vi "WPI_CANTalonSRX_ConfigEnabledLimits.vi"(0 "CAN Talon SRX Ref":T1={"DeviceStatus"={"status"=FALSE, "code"=0, "source"=""}, "Type"=enum."PWM", "PWM"={"PWM Channel"=enum."PWM 1", "DeadBand"={"Name"="", "maxPositivePwm"=0, "minPositivePwm"=0, "centerPwm"=0, "maxNegativePwm"=0, "minNegativePwm"=0, "angularRange"=0}}, "CAN"={"Device Number"=0, "SetOutput VI Ref"=variant(enum8{"Percent VBus", "Current", "Speed", "Position", "Voltage"} enum."Percent VBus"), "GetOutput VI Ref"=variant(refnum<k1> refnum), "Enable VI Ref"=variant(dbl 12.0), "Disable VI Ref"=variant(enum8{"Percent VBus", "Speed", "Position", "Slave", "Unchanged / Invalid", "Voltage Compensation", "Current", "Motion Profile"} enum."Percent VBus"), "Data"=variant}, "Invert"=FALSE}, 5 "Override Limit Switches":bool, 7 "Forward Limit Switch Enable":bool=TRUE, 9 "Reverse Limit Switch Enable":bool=TRUE, 11 "error in (no error)":errorcluster, 12 "Forward Soft Limit Enable":bool, 13 "Reverse Soft Limit Enable":bool) -> (4 "CAN Talon SRX Ref":T1={"DeviceStatus"={"status"=FALSE, "code"=0, "source"=""}, "Type"=enum."PWM", "PWM"={"PWM Channel"=enum."PWM 1", "DeadBand"={"Name"="", "maxPositivePwm"=0, "minPositivePwm"=0, "centerPwm"=0, "maxNegativePwm"=0, "minNegativePwm"=0, "angularRange"=0}}, "CAN"={"Device Number"=0, "SetOutput VI Ref"=variant(enum8{"Percent VBus", "Current", "Speed", "Position", "Voltage"} enum."Percent VBus"), "GetOutput VI Ref"=variant(refnum<k1> refnum), "Enable VI Ref"=variant(dbl 12.0), "Disable VI Ref"=variant(enum8{"Percent VBus", "Speed", "Position", "Slave", "Unchanged / Invalid", "Voltage Compensation", "Current", "Motion Profile"} enum."Percent VBus"), "Data"=variant}, "Invert"=FALSE}, 15 "error out":errorcluster)   [LabVIEW 2016]
doc: "Configure the enable state of the hardware limit switches and the soft limits."
uses:
  <vilib>/Rock Robotics/WPI/MotorControl/WPI_MotorControlDeviceRef.ctl
  <vilib>/Rock Robotics/WPI/MotorControl/WPI_MotorControlType.ctl
  <vilib>/Rock Robotics/SystemInterfaces/DIO/FPGA_DIOPWMChannel.ctl
  <vilib>/Rock Robotics/WPI/PWM/WPI_PWMDeadband.ctl
  <vilib>/Rock Robotics/WPI/ThirdParty/CanMotor/TalonSRX/WPI_CANTalonSRX_GlobalOps.ctl
  <vilib>/Rock Robotics/WPI/ThirdParty/CanMotor/TalonSRX/WPI_CANTalonSRX_Params.ctl
  <vilib>/Rock Robotics/WPI/ThirdParty/CanMotor/TalonSRX/CTRE_CANTalonSRX_UsageTypes.ctl
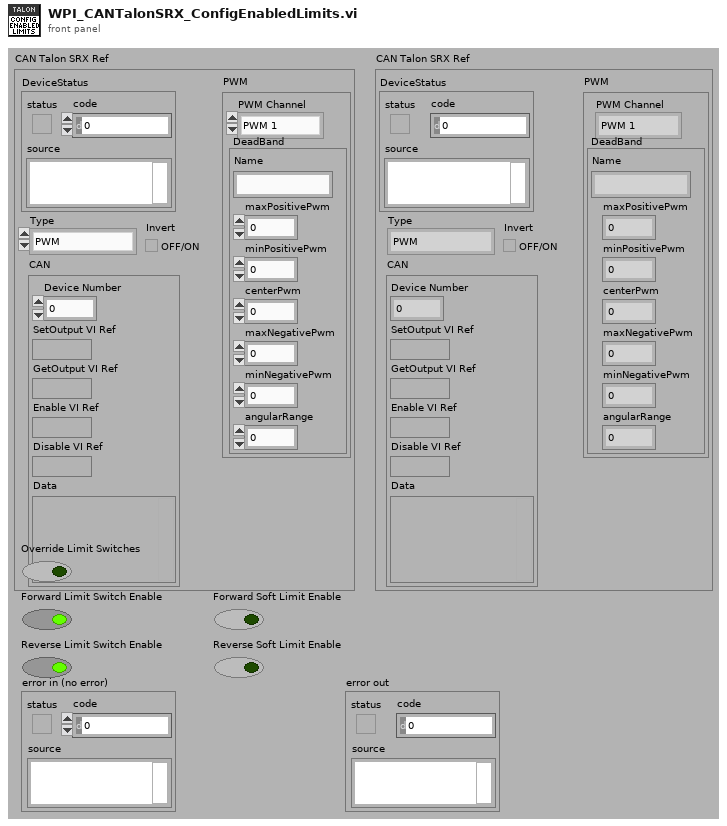
[diagram p1: front panel]
types:
  T1 = typedef "WPI_MotorControlDeviceRef.ctl" = cluster{"DeviceStatus":errorcluster, "Type":T2, "PWM":cluster{"PWM Channel":T3, "DeadBand":T4}, "CAN":cluster{"Device Number":u8, "SetOutput VI Ref":variant, "GetOutput VI Ref":variant, "Enable VI Ref":variant, "Disable VI Ref":variant, "Data":variant}, "Invert":bool}
  T2 = typedef "WPI_MotorControlType.ctl" = enum16{"PWM", "CAN"}
  T3 = typedef "FPGA_DIOPWMChannel.ctl" = enum8{"PWM 0", "PWM 1", "PWM 2", "PWM 3", "PWM 4", "PWM 5", "PWM 6", "PWM 7", "PWM 8", "PWM 9", "PWM MXP 0", "PWM MXP 1", "PWM MXP 2", "PWM MXP 3", "PWM MXP 4", "PWM MXP 5", "PWM MXP 6", "PWM MXP 7", "PWM MXP 8", "PWM MXP 9", "Invalid"}
  T4 = typedef "WPI_PWMDeadband.ctl" = cluster{"Name":string, "maxPositivePwm":i32, "minPositivePwm":i32, "centerPwm":i32, "maxNegativePwm":i32, "minNegativePwm":i32, "angularRange":u16}
  T5 = typedef "WPI_CANTalonSRX_GlobalOps.ctl" = enum16{"Read For Send", "Write After Receive General", "Write After Receive Feedback", "Write After Receive Encoder", "Write After Receive Ain", "Write Error", "Get All", "Set Output", "Set Mode", "Set Master ID", "Set Brake Mode", "Set Reverse Feedback Sensor", "Set Reverse Closed Loop Output", "Set Override Limits", "Set Forward Limit Enabled", "Set Reverse Limit Enabled", "Set Feedback Select", "Set Profile Select", "Set Throttle Ramp Rate", "Disable", "Set Enc Codes Per Rev", "Set Num Pot Turns", "Set Control Frame Rate", "Enable Legacy Control", "Write After Receive Pulse Width", "Set Enable Frame Rate", "Write After Receive Motion Profile", "Set Motion Profile Flow Control", "Set Motion Profile Control Frame Rate", "Set Current Limit Enable", "Set Usage Frame"}
  T6 = typedef "WPI_CANTalonSRX_Params.ctl" = u8
  T7 = typedef "CTRE_CANTalonSRX_UsageTypes.ctl" = u32
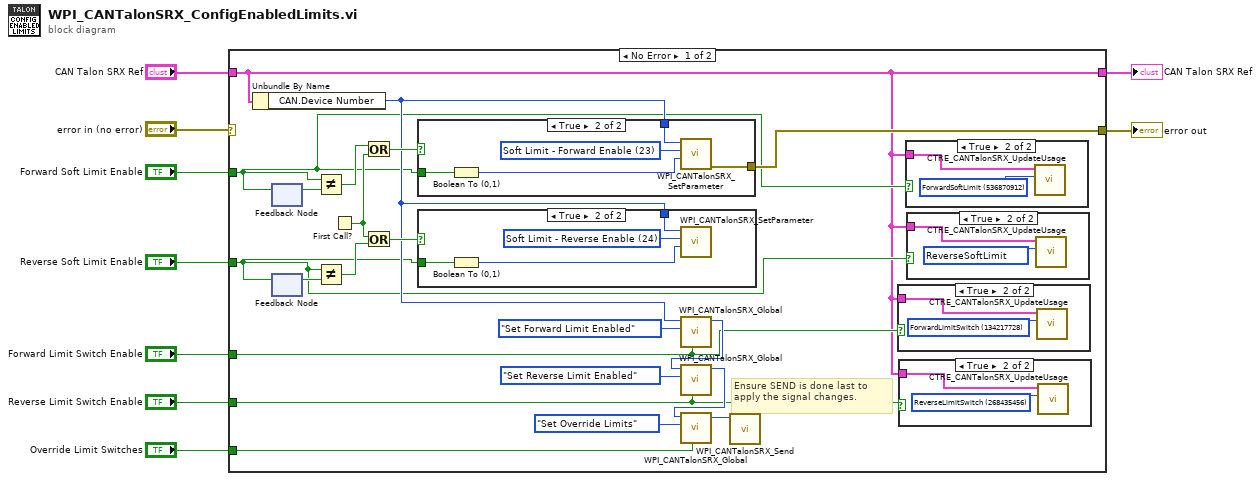
[diagram p0: block diagram]
diagram:
  n1 = case shown="No Error" "error in (no error)" {
    selector: "error in (no error)" -> [_ w49]
    tunnel: [w30 w49] -> w9
    tunnel: [w10 w48] -> w7
    tunnel: "CAN Talon SRX Ref" -> [w10 w48]
    tunnel: "Reverse Soft Limit Enable" -> [w13 _]
    tunnel: "Forward Soft Limit Enable" -> [w14 _]
    tunnel: "Reverse Limit Switch Enable" -> [w11 _]
    tunnel: "Forward Limit Switch Enable" -> [w12 _]
    tunnel: "Override Limit Switches" -> [w27 _]
    frame No Error {
      # "Ensure SEND is done last to apply the signal changes."
      n2 = Unbundle By Name(w10) -> ("CAN.Device Number"=w18:u8)
      n3 = feedback #1() -> (w21:bool)  [unwired: 1 in]
      n4 = feedback-in #1(w14) -> ()
      n5 = feedback-in #2(w13) -> ()
      n6 = feedback #2() -> (w25:bool)  [unwired: 1 in]
      n7 = Not Equal?(x=w14, y=w21) -> (x != y?=w22:bool)
      n8 = Not Equal?(x=w13, y=w25) -> (x != y?=w23:bool)
      n9 = First Call?() -> (First Call?: T/F=w20:bool)
      n10 = Or(x=w22, y=w20) -> (x .or. y?=w19:bool)
      n11 = Or(x=w20, y=w23) -> (x .or. y?=w24:bool)
      n12 = case shown="True" w19 {
        tunnel: w14 -> [_ w42]
        tunnel: [_ w40] -> w30
        tunnel: w18 -> [_ w39]
        frame False {
        }
        frame True {
          w43 = T6 23 items=["Slot 0 - P"=1, "Slot 0 - I"=2, "Slot 0 - D"=3, "Slot 0 - F"=4, "Slot 0 - I Zone"=5, "Slot 0 - Ramp Rate"=6, "Slot 1 - P"=11, "Slot 1 - I"=12, "Slot 1 - D"=13, "Slot 1 - F"=14, "Slot 1 - I Zone"=15, "Slot 1 - Ramp Rate"=16, "Soft Limit - Forward"=21, "Soft Limit - Reverse"=22, "Soft Limit - Forward Enable"=23, "Soft Limit - Reverse Enable"=24, "On Boot - Brake Mode"=31, "On Boot - Limit Normally Closed - Forward"=32, "On Boot - Limit Normally Closed - Reverse"=33, "On Boot - Limit Disabled - Forward"=34, "On Boot - Limit Disabled - Reverse"=35, "Fault - Over Temp"=41, "Fault - Under Voltage"=42, "Fault - Forward Limit"=43, "Fault - Reverse Limit"=44, "Fault - Hardware Failure"=45, "Fault - Forward Soft Limit"=46, "Fault - Reverse Soft Limit"=47, "Sticky Fault - Over Temp"=48, "Sticky Fault - Under Voltage"=49, "Sticky Fault - Forward Limit"=50, "Sticky Fault - Reverse Limit"=51, "Sticky Fault - Forward Soft Limit"=52, "Sticky Fault - Reverse Soft Limit"=53, "Applied Throttle"=61, "Closed-Loop Error"=62, "Select Feedback Device"=63, "Reverse Closed-Loop Output"=64, "Mode Select"=65, "Profile Slot Select"=66, "Ramp Throttle"=67, "Reverse Feedback Sensor"=68, "Limit Switch Enabled"=69, "Limit Switch Closed - Forward"=70, "Limit Switch Closed - Reverse"=71, "Sensor Position"=73, "Sensor Velocity"=74, "Current"=75, "Brake is Enabled"=76, "Encoder Position"=77, "Encoder Velocity"=78, "Encoder Index Rise Events"=79, "Encoder A Pin State"=80, "Encoder B Pin State"=81, "Encoder Index Pin State"=82, "Analog In with Overflow"=83, "Analog In Velocity"=84, "Temperature"=85, "Battery Voltage"=86, "Reset Count"=87, "Reset Flags"=88, "Firmware Version"=89, "Settings Changed"=90] ("Parameter")
          n13 = Boolean To (0,1)(Boolean=w42) -> (0, 1=w41:i16)
          n14 = call <vilib>:"WPI_CANTalonSRX_SetParameter.vi"("Value"=w41, "Parameter"=w43, "Device ID (0)"=w39) -> ("error out"=w40:errorcluster)  [unwired: 7 in, 1 out]
        }
      }
      n15 = case shown="True" w24 {
        tunnel: w13 -> [_ w46]
        tunnel: w18 -> [_ w44]
        frame False {
        }
        frame True {
          w47 = T6 24 items=["Slot 0 - P"=1, "Slot 0 - I"=2, "Slot 0 - D"=3, "Slot 0 - F"=4, "Slot 0 - I Zone"=5, "Slot 0 - Ramp Rate"=6, "Slot 1 - P"=11, "Slot 1 - I"=12, "Slot 1 - D"=13, "Slot 1 - F"=14, "Slot 1 - I Zone"=15, "Slot 1 - Ramp Rate"=16, "Soft Limit - Forward"=21, "Soft Limit - Reverse"=22, "Soft Limit - Forward Enable"=23, "Soft Limit - Reverse Enable"=24, "On Boot - Brake Mode"=31, "On Boot - Limit Normally Closed - Forward"=32, "On Boot - Limit Normally Closed - Reverse"=33, "On Boot - Limit Disabled - Forward"=34, "On Boot - Limit Disabled - Reverse"=35, "Fault - Over Temp"=41, "Fault - Under Voltage"=42, "Fault - Forward Limit"=43, "Fault - Reverse Limit"=44, "Fault - Hardware Failure"=45, "Fault - Forward Soft Limit"=46, "Fault - Reverse Soft Limit"=47, "Sticky Fault - Over Temp"=48, "Sticky Fault - Under Voltage"=49, "Sticky Fault - Forward Limit"=50, "Sticky Fault - Reverse Limit"=51, "Sticky Fault - Forward Soft Limit"=52, "Sticky Fault - Reverse Soft Limit"=53, "Applied Throttle"=61, "Closed-Loop Error"=62, "Select Feedback Device"=63, "Reverse Closed-Loop Output"=64, "Mode Select"=65, "Profile Slot Select"=66, "Ramp Throttle"=67, "Reverse Feedback Sensor"=68, "Limit Switch Enabled"=69, "Limit Switch Closed - Forward"=70, "Limit Switch Closed - Reverse"=71, "Sensor Position"=73, "Sensor Velocity"=74, "Current"=75, "Brake is Enabled"=76, "Encoder Position"=77, "Encoder Velocity"=78, "Encoder Index Rise Events"=79, "Encoder A Pin State"=80, "Encoder B Pin State"=81, "Encoder Index Pin State"=82, "Analog In with Overflow"=83, "Analog In Velocity"=84, "Temperature"=85, "Battery Voltage"=86, "Reset Count"=87, "Reset Flags"=88, "Firmware Version"=89, "Settings Changed"=90] ("Parameter")
          n16 = Boolean To (0,1)(Boolean=w46) -> (0, 1=w45:i16)
          n17 = call <vilib>:"WPI_CANTalonSRX_SetParameter.vi"("Value"=w45, "Parameter"=w47, "Device ID (0)"=w44) -> ()  [unwired: 7 in, 2 out]
        }
      }
      n18 = call <vilib>:"WPI_CANTalonSRX_Global.vi"("Set Boolean"=w12, "Operation"=WPI_CANTalonSRX_GlobalOps."Set Forward Limit Enabled", "Device ID (0)"=w18) -> ("Device ID Out"=w16:u8)  [unwired: 6 in, 2 out]
      n19 = call <vilib>:"WPI_CANTalonSRX_Global.vi"("Set Boolean"=w11, "Operation"=WPI_CANTalonSRX_GlobalOps."Set Reverse Limit Enabled", "Device ID (0)"=w16) -> ("Device ID Out"=w15:u8)  [unwired: 6 in, 2 out]
      n20 = call <vilib>:"WPI_CANTalonSRX_Global.vi"("Set Boolean"=w27, "Operation"=WPI_CANTalonSRX_GlobalOps."Set Override Limits", "Device ID (0)"=w15) -> ("Device ID Out"=w17:u8)  [unwired: 6 in, 2 out]
      n21 = call <vilib>:"WPI_CANTalonSRX_Send.vi"("Device ID (0)"=w17) -> ()  [unwired: 10 in, 1 out]
      n22 = case shown="True" w12 {
        tunnel: w10 -> [_ w34]
        frame False {
        }
        frame True {
          w33 = T7 134217728 items=["Default"=0, "PercentVbus"=1, "Position"=2, "Speed"=4, "Current"=8, "Voltage"=16, "Follower"=32, "MotionProfile"=64, "MotionMagic"=128, "VRampRate"=4194304, "CurrentLimit"=8388608, "ZeroSensorI"=16777216, "ZeroSensorF"=33554432, "ZeroSensorR"=67108864, "ForwardLimitSwitch"=134217728, "ReverseLimitSwitch"=268435456, "ForwardSoftLimit"=536870912, "ReverseSoftLimit"=1073741824, "MultiProfile"=2147483648] ("Usage")
          n23 = call <vilib>:"CTRE_CANTalonSRX_UpdateUsage.vi"("Usage"=w33, "CAN Talon SRX Ref"=w34) -> ()  [unwired: 10 in]
        }
      }
      n24 = case shown="True" w11 {
        tunnel: w10 -> [_ w32]
        frame False {
        }
        frame True {
          w31 = T7 268435456 items=["Default"=0, "PercentVbus"=1, "Position"=2, "Speed"=4, "Current"=8, "Voltage"=16, "Follower"=32, "MotionProfile"=64, "MotionMagic"=128, "VRampRate"=4194304, "CurrentLimit"=8388608, "ZeroSensorI"=16777216, "ZeroSensorF"=33554432, "ZeroSensorR"=67108864, "ForwardLimitSwitch"=134217728, "ReverseLimitSwitch"=268435456, "ForwardSoftLimit"=536870912, "ReverseSoftLimit"=1073741824, "MultiProfile"=2147483648] ("Usage")
          n25 = call <vilib>:"CTRE_CANTalonSRX_UpdateUsage.vi"("Usage"=w31, "CAN Talon SRX Ref"=w32) -> ()  [unwired: 10 in]
        }
      }
      n26 = case shown="True" w14 {
        tunnel: w10 -> [_ w38]
        frame False {
        }
        frame True {
          w37 = T7 536870912 items=["Default"=0, "PercentVbus"=1, "Position"=2, "Speed"=4, "Current"=8, "Voltage"=16, "Follower"=32, "MotionProfile"=64, "MotionMagic"=128, "VRampRate"=4194304, "CurrentLimit"=8388608, "ZeroSensorI"=16777216, "ZeroSensorF"=33554432, "ZeroSensorR"=67108864, "ForwardLimitSwitch"=134217728, "ReverseLimitSwitch"=268435456, "ForwardSoftLimit"=536870912, "ReverseSoftLimit"=1073741824, "MultiProfile"=2147483648] ("Usage")
          n27 = call <vilib>:"CTRE_CANTalonSRX_UpdateUsage.vi"("Usage"=w37, "CAN Talon SRX Ref"=w38) -> ()  [unwired: 10 in]
        }
      }
      n28 = case shown="True" w13 {
        tunnel: w10 -> [_ w36]
        frame False {
        }
        frame True {
          w35 = T7 1073741824 items=["Default"=0, "PercentVbus"=1, "Position"=2, "Speed"=4, "Current"=8, "Voltage"=16, "Follower"=32, "MotionProfile"=64, "MotionMagic"=128, "VRampRate"=4194304, "CurrentLimit"=8388608, "ZeroSensorI"=16777216, "ZeroSensorF"=33554432, "ZeroSensorR"=67108864, "ForwardLimitSwitch"=134217728, "ReverseLimitSwitch"=268435456, "ForwardSoftLimit"=536870912, "ReverseSoftLimit"=1073741824, "MultiProfile"=2147483648] ("Usage")
          n29 = call <vilib>:"CTRE_CANTalonSRX_UpdateUsage.vi"("Usage"=w35, "CAN Talon SRX Ref"=w36) -> ()  [unwired: 10 in]
        }
      }
    }
    frame Error {
    }
  }
  "CAN Talon SRX Ref" <- w7
  "error out" <- w9
